vi "Minda Time Lock.vi"(8 "error in":errorcluster) -> (0 "error out":errorcluster, 3 "Time Laps":bool)   [LabVIEW 2017]
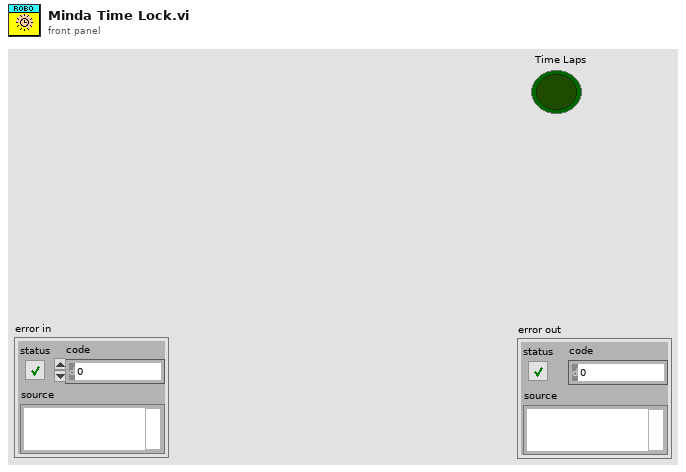
[diagram p1: front panel]
types:
  T1 = typedef "LVDateTimeRec.ctl" = cluster{"fractional second":dbl, "second":i32, "minute":i32, "hour":i32, "day of month":i32, "month":i32, "year":i32, "day of week":i32, "day of year":i32, "DST":i32}
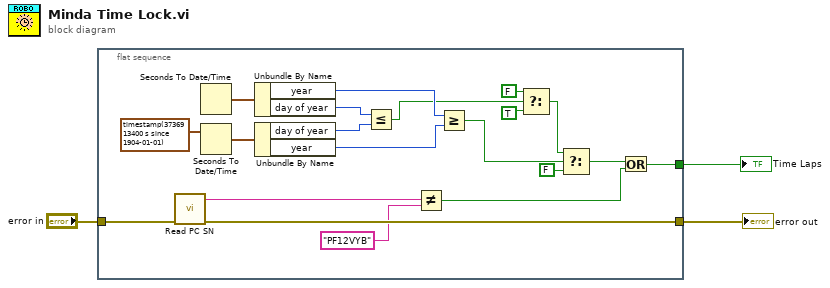
[diagram p0: block diagram]
diagram:
  n1 = flat-sequence {
    tunnel: [w6] -> w1
    tunnel: "error in" -> [w9]
    tunnel: [w8] -> w2
    frame #0 {
      n2 = call "Read PC SN.vi"("error in (no error)"=w9) -> ("error out"=w8:errorcluster, "Serial Number"=w7:string)  [unwired: 9 in]
      n3 = Seconds To Date/Time() -> (date time rec=w21:T1)  [unwired: 2 in]
      n4 = Seconds To Date/Time(time stamp (now)=timestamp(3736913400 s since 1904-01-01) ("time stamp")) -> (date time rec=w23:T1)  [unwired: 1 in]
      n5 = Unbundle By Name(w21) -> ("year"=w20:i32, "day of year"=w13:i32)
      n6 = Unbundle By Name(w23) -> ("day of year"=w12:i32, "year"=w19:i32)
      n7 = Less Or Equal?(x=w13, y=w12) -> (x <= y?=w11:bool)
      n8 = Not Equal?(x=w7, y="PF12VYB") -> (x != y?=w5:bool)
      n9 = Greater Or Equal?(x=w20, y=w19) -> (x >= y?=w14:bool)
      n10 = Select(t=FALSE, s=w11, f=TRUE) -> (s? t:f=w17:bool)
      n11 = Select(t=w17, s=w14, f=FALSE) -> (s? t:f=w15:bool)
      n12 = Or(x=w15, y=w5) -> (x .or. y?=w6:bool)
    }
  }
  "Time Laps" <- w1
  "error out" <- w2
